vi "Buttons to Message-Simple.vi"(9 "Down Button":bool, 10 "Stop Button":bool, 11 "Up Button":bool) -> (3 "Control Word":string)   [LabVIEW 2021]
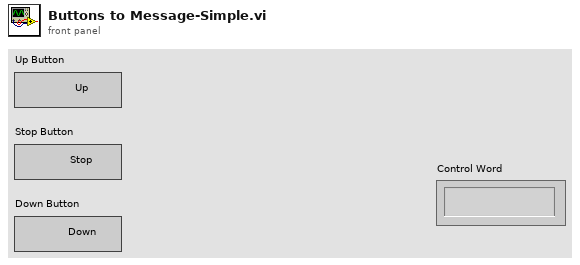
[diagram p1: front panel]
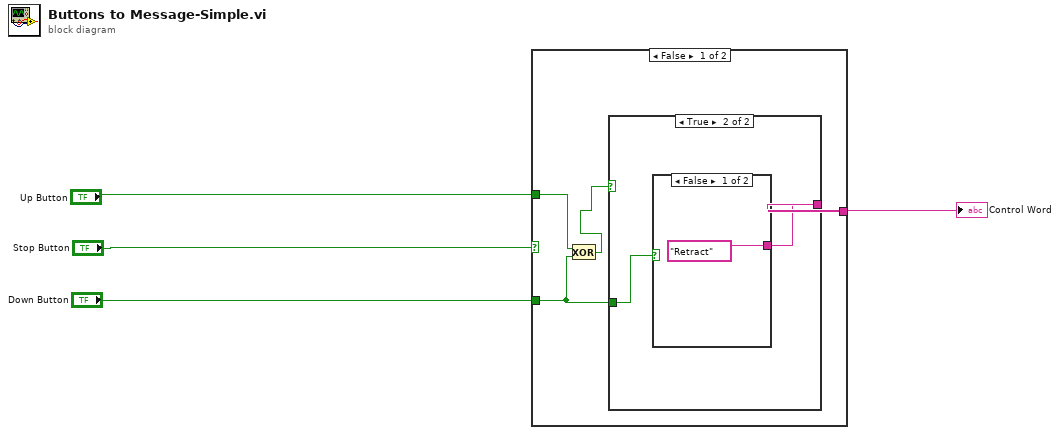
[diagram p0: block diagram]
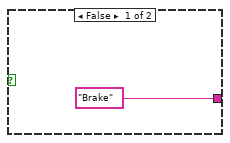
[diagram p2: hidden frame]
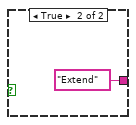
[diagram p3: hidden frame]
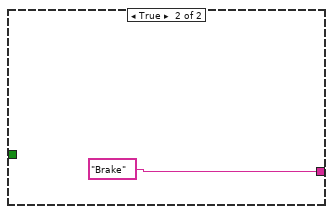
[diagram p4: hidden frame]
diagram:
  n1 = case shown="False" "Stop Button" {
    tunnel: [w8 "Brake"] -> w4
    tunnel: "Up Button" -> [w7 _]
    tunnel: "Down Button" -> [w5 _]
    frame False {
      n2 = Exclusive Or(1:w5, 2:w7) -> (0:w6:bool)
      n3 = case shown="True" w6 {
        tunnel: ["Brake" w11] -> w8
        tunnel: w5 -> [_ w10]
        frame False {
        }
        frame True {
          n4 = case shown="False" w10 {
            tunnel: ["Retract" "Extend"] -> w11
            frame False {
            }
            frame True {
            }
          }
        }
      }
    }
    frame True {
    }
  }
  "Control Word" <- w4
